vi "OnDrop.vi"(0 "XRef":T16, 1 "State In":T1={"Worker Library Path"=path "", "Block Label"="", "Types"=[], "Selections"=[], "Icon"={"image type"=0, "image depth"=0, "image"=[], "mask"=[], "colors"=[], "Rectangle"={"left"=0, "top"=0, "right"=0, "bottom"=0}}, "Errors"={"Terminals"=[], "Generate"={"status"=FALSE, "code"=0, "source"=""}, "General"={"status"=FALSE, "code"=0, "source"=""}}, "Calculated Sizes"={"Block Width"=0, "Block Height"=0, "Half Width"=0, "Icon Top"=0, "Icon Bottom"=0, "Label Width"=0, "Half Label"=0, "Label Top"=0, "Text Width"=0, "Half Text"=0, "Text Height"=0, "Label Height"=0, "Expanded Width"=0, "Label Bottom"=0, "Expanded Top"=0, "Expanded Bottom"=0, "Expanded Height"=0, "Min Height"=0, "Max Height"=0}, "Special Terminal Indices"={"Action"=-1, "Init"=-1, "Tag"=-1, "State in"=-1, "State out"=-1, "Error"=-1}, "Terminals"=[]}) -> (14 "Reply":T14, 15 "Fatal Error Out":T13, 16 "State Out":T1={"Worker Library Path"=path "", "Block Label"="", "Types"=[], "Selections"=[], "Icon"={"image type"=0, "image depth"=0, "image"=[], "mask"=[], "colors"=[], "Rectangle"={"left"=0, "top"=0, "right"=0, "bottom"=0}}, "Errors"={"Terminals"=[], "Generate"={"status"=FALSE, "code"=0, "source"=""}, "General"={"status"=FALSE, "code"=0, "source"=""}}, "Calculated Sizes"={"Block Width"=0, "Block Height"=0, "Half Width"=0, "Icon Top"=0, "Icon Bottom"=0, "Label Width"=0, "Half Label"=0, "Label Top"=0, "Text Width"=0, "Half Text"=0, "Text Height"=0, "Label Height"=0, "Expanded Width"=0, "Label Bottom"=0, "Expanded Top"=0, "Expanded Bottom"=0, "Expanded Height"=0, "Min Height"=0, "Max Height"=0}, "Special Terminal Indices"={"Action"=-1, "Init"=-1, "Tag"=-1, "State in"=-1, "State out"=-1, "Error"=-1}, "Terminals"=[]})   [LabVIEW 2022 SP3, in "Flex Block.xnode"]
uses:
  Flex Block.xnode
  <vilib>/XNodeSupport/XNodeXNodeRef.ctl
  State.ctl
  FlexBlocks Support/Type Descriptor.ctl
  FlexBlocks Support/Terminal Direction.ctl
  FlexBlocks Support/Value Mode.ctl
  FlexBlocks Support/Special Terminal.ctl
  <vilib>/picture/picture.llb/imagedata.ctl
  FlexBlocks Support/XNode Errors.ctl
  FlexBlocks Support/Calculated Sizes.ctl
  FlexBlocks Support/Special Terminal Indices.ctl
  FlexBlocks Support/Terminal Status.ctl
  FlexBlocks Support/Terminal State.ctl
  FlexBlocks Support/Terminal Draw Style.ctl
  <vilib>/XNodeSupport/XNodeStringArray.ctl
  <vilib>/XNodeSupport/XNodeString.ctl
  <vilib>/XNodeSupport/XNodeErrorCluster.ctl
  FlexBlocks Support/FlexBlocks Support.lvlib
  <vilib>/XNodeSupport/NI_XNodeSupport.lvlib
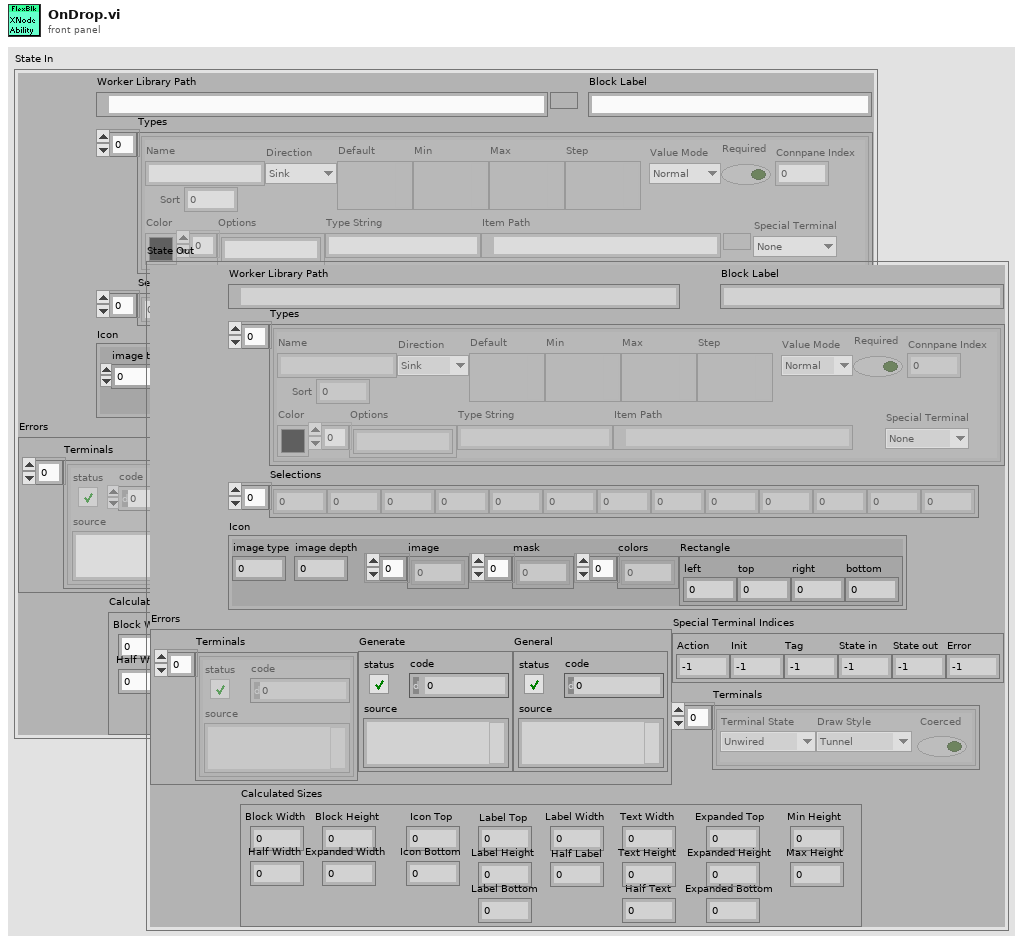
[diagram p1: front panel]
types:
  T1 = typedef "Flex Block.xnode/State.ctl" = cluster{"Worker Library Path":path, "Block Label":string, "Types":T2[], "Selections":i32[], "Icon":T6, "Errors":T7, "Calculated Sizes":T8, "Special Terminal Indices":T9, "Terminals":T10[]}
  T2 = typedef "FlexBlocks Support.lvlib/Type Descriptor.ctl" = cluster{"Name":string, "Direction":T3, "Default":variant, "Min":variant, "Max":variant, "Step":variant, "Value Mode":T4, "Color":u32, "Options":string[], "Type String":string, "Item Path":path, "Required":bool, "Connpane Index":i32, "Special Terminal":T5, "Sort":i32}
  T3 = typedef "FlexBlocks Support.lvlib/Terminal Direction.ctl" = enum16{"Sink", "Source"}
  T4 = typedef "FlexBlocks Support.lvlib/Value Mode.ctl" = enum16{"Normal", "Range", "Select"}
  T5 = typedef "FlexBlocks Support.lvlib/Special Terminal.ctl" = enum16{"None", "Action", "Init", "Tag", "State in", "State out", "Error"}
  T6 = typedef "imagedata.ctl" = cluster{"image type":i32, "image depth":i32, "image":u8[], "mask":u8[], "colors":u32[], "Rectangle":cluster{"left":i16, "top":i16, "right":i16, "bottom":i16}}
  T7 = typedef "FlexBlocks Support.lvlib/XNode Errors.ctl" = cluster{"Terminals":errorcluster[], "Generate":errorcluster, "General":errorcluster}
  T8 = typedef "FlexBlocks Support.lvlib/Calculated Sizes.ctl" = cluster{"Block Width":i32, "Block Height":i32, "Half Width":i32, "Icon Top":i32, "Icon Bottom":i32, "Label Width":i32, "Half Label":i32, "Label Top":i32, "Text Width":i32, "Half Text":i32, "Text Height":i32, "Label Height":i32, "Expanded Width":i32, "Label Bottom":i32, "Expanded Top":i32, "Expanded Bottom":i32, "Expanded Height":i32, "Min Height":i32, "Max Height":i32}
  T9 = typedef "FlexBlocks Support.lvlib/Special Terminal Indices.ctl" = cluster{"Action":i32, "Init":i32, "Tag":i32, "State in":i32, "State out":i32, "Error":i32}
  T10 = typedef "FlexBlocks Support.lvlib/Terminal Status.ctl" = cluster{"Terminal State":T11, "Draw Style":T12, "Coerced":bool}
  T11 = typedef "FlexBlocks Support.lvlib/Terminal State.ctl" = enum16{"Unwired", "BadType", "BadRef", "Channel", "Value", "Control Ref"}
  T12 = typedef "FlexBlocks Support.lvlib/Terminal Draw Style.ctl" = enum16{"Tunnel", "BadType", "BadRef", "Channel", "Value", "Control Ref"}
  T13 = typedef "NI_XNodeSupport.lvlib/XNodeErrorCluster.ctl" = errorcluster
  T14 = typedef "NI_XNodeSupport.lvlib/XNodeStringArray.ctl" = T15[]
  T15 = typedef "NI_XNodeSupport.lvlib/XNodeString.ctl" = string
  T16 = typedef "NI_XNodeSupport.lvlib/XNodeXNodeRef.ctl" = refnum<vi>
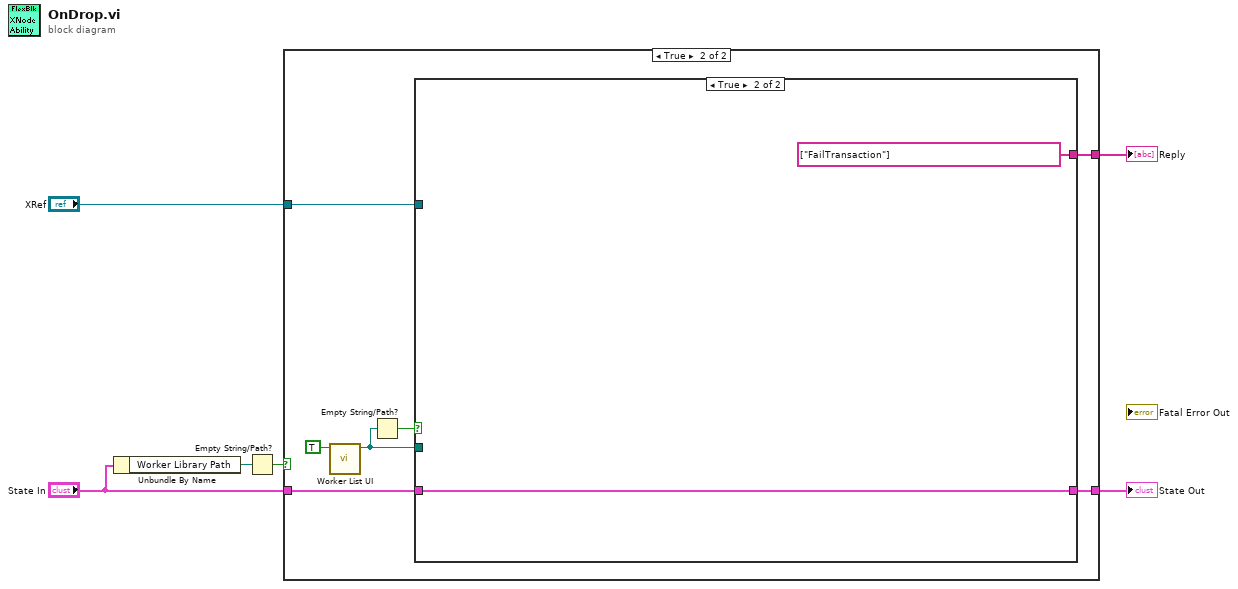
[diagram p0: block diagram]
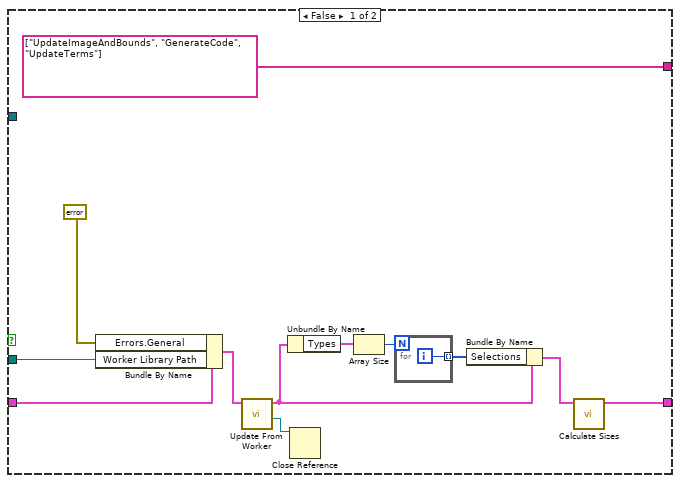
[diagram p3: hidden frame]
diagram:
  n1 = Unbundle By Name("State In") -> ("Worker Library Path"=w3:path)
  n2 = Empty String/Path?(string/path=w3) -> (empty?=w2:bool)
  n3 = case shown="True" w2 {
    tunnel: "State In" -> [w7 w13]
    tunnel: [w7 w10] -> w5
    tunnel: [_ w9] -> w4
    tunnel: "XRef" -> [_ w8]
    frame False {
    }
    frame True {
      n4 = call "Worker List UI.vi"("Opened from Block"=TRUE) -> ("Selected Worker Lib"=w11:path)  [unwired: 10 in]
      n5 = Empty String/Path?(string/path=w11) -> (empty?=w12:bool)
      n6 = case shown="True" w12 {
        tunnel: w13 -> [w26 w29]
        tunnel: w11 -> [w25 _]
        tunnel: [w15 w29] -> w10
        tunnel: [T14 ["UpdateImageAndBounds", "GenerateCode", "UpdateTerms"] ("Reply") T14 ["FailTransaction"] ("Reply")] -> w9
        tunnel: w8 -> [_ _]
        frame False {
          n7 = Bundle By Name(cluster=w26, "Errors.General"=errorcluster {"status"=FALSE, "code"=0, "source"=""}, "Worker Library Path"=w25) -> (w23:T1)
          n8 = call "Update From Worker.vi"("State In"=w23) -> ("Worker VI"=w22:refnum<vi>, "State"=w17:T1)  [unwired: 9 in]
          n9 = Unbundle By Name(w17) -> ("Types"=w20:T2[])
          n10 = Close Reference(reference=w22) -> ()  [unwired: 1 in, 1 out]
          n11 = Array Size(array=w20) -> (size(s)=w19:i32)
          n12 = for {
            N: w19 -> [_]
            tunnel: [w27] -> w18 mode=indexing
            i -> [w27]
          }
          n13 = Bundle By Name(cluster=w17, "Selections"=w18) -> (w16:T1)
          n14 = call "Calculate Sizes.vi"("State In"=w16) -> ("State"=w15:T1)  [unwired: 10 in]
        }
        frame True {
        }
      }
    }
  }
  "Reply" <- w4
  "State Out" <- w5
